vi "数组非0值的均值子VI.vi"(2 "数组":dbl[](array[numeric])) -> (0 "平均值":dbl)   [LabVIEW 2013]
panel:
  in  "不为0的数个数":dbl
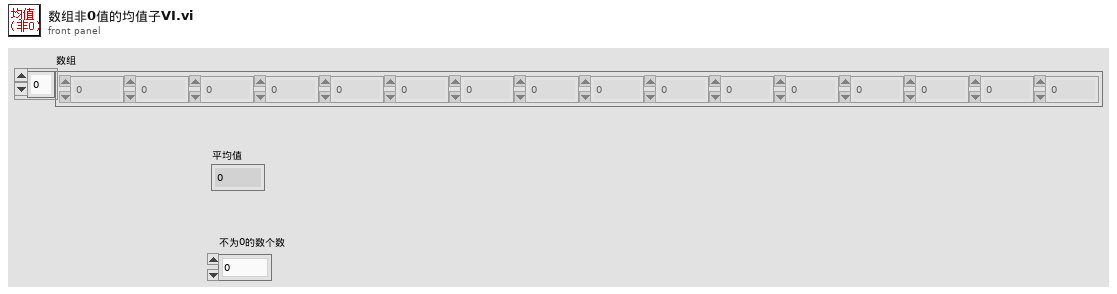
[diagram p1: front panel]
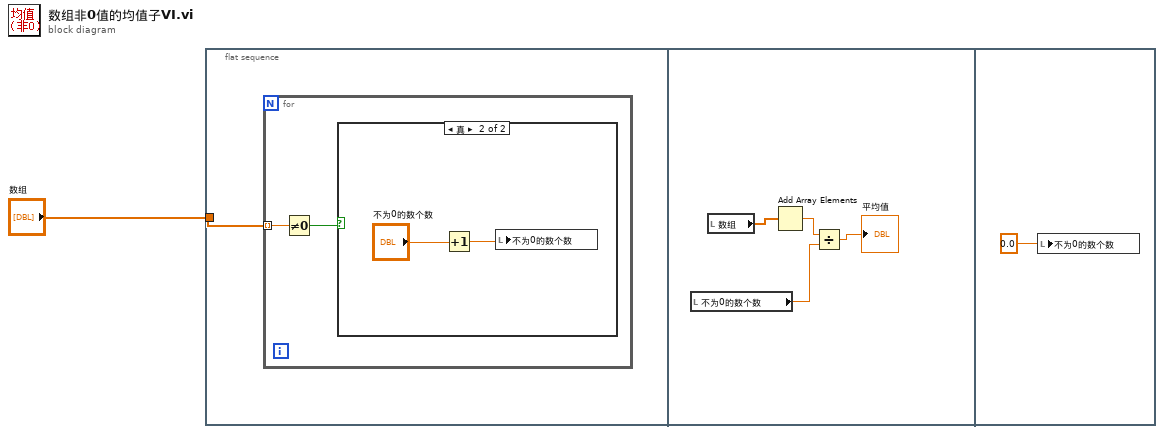
[diagram p0: block diagram]
diagram:
  n1 = flat-sequence {
    tunnel: "数组" -> [w2]
    frame #0 {
      n2 = for {
        tunnel: w2 -> [w3] mode=indexing
        n3 = Not Equal To 0?(x=w3) -> (x != 0?=w4:bool)
        n4 = case shown="真" w4 {
          frame False {
          }
          frame True {
            n5 = Increment(x="不为0的数个数") -> (x+1=w5:dbl)
            n6 = local write "不为0的数个数"(w5) -> ()
          }
        }
      }
    }
    frame #1 {
      n7 = local read "不为0的数个数"() -> (w7:dbl)
      n8 = local read "数组"() -> (w10:dbl[])
      n9 = Add Array Elements(numeric array=w10) -> (sum=w9:dbl)
      n10 = Divide(x=w9, y=w7) -> (x/y=→"平均值":dbl)
    }
    frame #2 {
      n11 = local write "不为0的数个数"(0.0 ("不为0的数个数")) -> ()
    }
  }
